vi "GetMatchTimestamp.vi"(8 "seconds since 1Jan1904":timestamp, 10 "Robot Mode":T1, 11 "Boolean":bool) -> (0 "seconds since 1Jan1904 2":timestamp, 2 "Match Timestamp":string)   [LabVIEW 2015]
uses:
  <vilib>/Rock Robotics/WPI/DriverStation/WPI_DriverStationRobotMode2.ctl
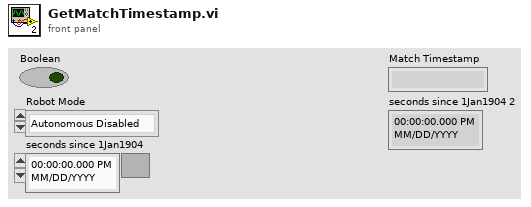
[diagram p1: front panel]
types:
  T1 = typedef "WPI_DriverStationRobotMode2.ctl" = enum16{"Autonomous Disabled", "Autonomous Enabled", "Teleop Disabled", "Teleop Enabled", "Disconnected", "Finish", "Test Disabled", "Test Enabled", "Emergency Stopped"}
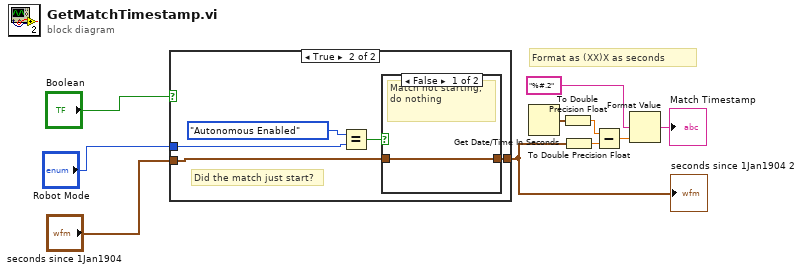
[diagram p0: block diagram]
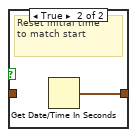
[diagram p3: hidden frame]
diagram:
  # "Format as (XX)X as seconds"
  n1 = case shown="True" "Boolean" {
    tunnel: "Robot Mode" -> [_ w14]
    tunnel: "seconds since 1Jan1904" -> [w11 w13]
    tunnel: [w11 w12] -> w2
    frame False {
    }
    frame True {
      # "Did the match just start?"
      n2 = Equal?(x=WPI_DriverStationRobotMode2."Autonomous Enabled" ("Robot Mode"), y=w14) -> (x = y?=w16:bool)
      n3 = case shown="False" w16 {
        tunnel: w13 -> [w17 _]
        tunnel: [w17 w18] -> w12
        frame False {
          # "Match not starting,\ndo nothing"
        }
        frame True {
          # "Reset initial time\nto match start"
          n4 = Get Date/Time In Seconds() -> (seconds since 1Jan1904=w18:timestamp)
        }
      }
    }
  }
  "seconds since 1Jan1904 2" <- w2
  n5 = Get Date/Time In Seconds() -> (seconds since 1Jan1904=w8:timestamp)
  n6 = To Double Precision Float(number=w8) -> (double precision float=w7:dbl)
  n7 = To Double Precision Float(number=w2) -> (double precision float=w6:dbl)
  n8 = Subtract(x=w7, y=w6) -> (x-y=w9:dbl)
  n9 = Format Value(format string="%#.2", value (0)=w9) -> (output string=→"Match Timestamp":string)  [unwired: 1 in]
